vi "AMZ_S3_ERR_Get Call Result.vi"(8 "error in (no error)":errorcluster, 11 "Response body":string) -> (0 "error out":errorcluster, 3 "Call Result":T1)   [LabVIEW 2015, in "LV Interface for Amazon S3.lvlib"]
uses:
  LV Interface for Amazon S3.lvlib
  Typedefs/AMZ_S3_Call Results.ctl
  <vilib>/regexp/Match Regular Expression.xnode
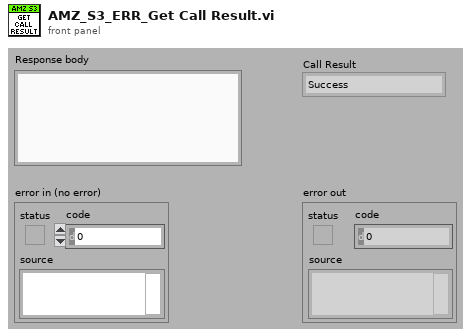
[diagram p1: front panel]
types:
  T1 = typedef "LV Interface for Amazon S3.lvlib/AMZ_S3_Call Results.ctl" = enum16{"Success", "UndefinedError", "AccessDenied", "AccountProblem", "AmbiguousGrantByEmailAddress", "BadDigest", "BucketAlreadyExists", "BucketAlreadyOwnedByYou", "BucketNotEmpty", "CredentialsNotSupported", "CrossLocationLoggingProhibited", "EntityTooSmall", "EntityTooLarge", "ExpiredToken", "IllegalVersioningConfigurationException", "IncompleteBody", "IncorrectNumberOfFilesInPostRequest", "InlineDataTooLarge", "InternalError", "InvalidAccessKeyId", "InvalidAddressingHeader", "InvalidArgument", "InvalidBucketName", "InvalidDigest", "InvalidLocationConstraint", "InvalidPart", "InvalidPartOrder", "InvalidPayer", "InvalidPolicyDocument", "InvalidRange", "InvalidSecurity", "InvalidSOAPRequest", "InvalidStorageClass", "InvalidTargetBucketForLogging", "InvalidToken", "InvalidURI", "KeyTooLong", "MalformedACLError", "MalformedPOSTRequest", "MalformedXML", "MaxMessageLengthExceeded", "MaxPostPreDataLengthExceededError", "MetadataTooLarge", "MethodNotAllowed", "MissingAttachment", "MissingContentLength", "MissingRequestBodyError", "MissingSecurityElement", "MissingSecurityHeader", "NoLoggingStatusForKey", "NoSuchBucket", "NoSuchKey", "NoSuchUpload", "NoSuchVersion", "NotImplemented", "NotSignedUp", "OperationAborted", "PermanentRedirect", "PreconditionFailed", "Redirect", "RequestIsNotMultiPartContent", "RequestTimeout", "RequestTimeTooSkewed", "RequestTorrentOfBucketError", "SignatureDoesNotMatch", "SlowDown", "TemporaryRedirect", "TokenRefreshRequired", "TooManyBuckets", "UnexpectedContent", "UnresolvableGrantByEmailAddress", "UserKeyMustBeSpecified", "LabVIEWError"}
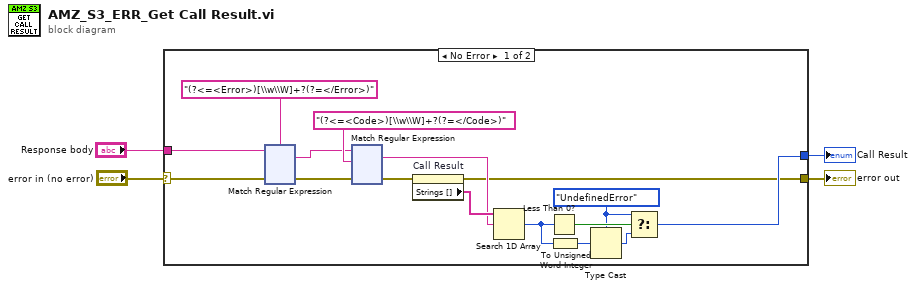
[diagram p0: block diagram]
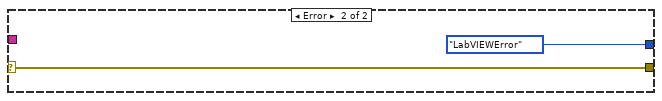
[diagram p2: hidden frame]
diagram:
  n1 = case shown="No Error" "error in (no error)" {
    selector: "error in (no error)" -> [w20 w250]
    tunnel: "Response body" -> [w19 _]
    tunnel: [w5 w250] -> w2
    tunnel: [w10 AMZ_S3_Call_Results."LabVIEWError" ("Call Result")] -> w1
    frame No Error {
      w7 = AMZ_S3_Call_Results."UndefinedError" ("Call Result")
      n2 = xnode "Match Regular Expression"("input string"=w19, "regular expression"="(?<=<Error>)[\\w\\W]+?(?=</Error>)", "error in"=w20) -> ("whole match"=w9:string, "error out"=w17:errorcluster)  [unwired: 3 in, 3 out]
      n3 = xnode "Match Regular Expression"("input string"=w9, "regular expression"="(?<=<Code>)[\\w\\W]+?(?=</Code>)", "error in"=w17) -> ("whole match"=w13:string, "error out"=w15:errorcluster)  [unwired: 3 in, 3 out]
      n4 = property on="Call Result" class="Enum (strict)"(error in=w15) -> (error out=w5:errorcluster, "Strings []"=w14:string[])  [unwired: 1 in, 1 out]
      n5 = Search 1D Array(1D array=w14, element=w13) -> (index of element=w11:i32)  [unwired: 1 in]
      n6 = Less Than 0?(x=w11) -> (x < 0?=w12:bool)
      n7 = To Unsigned Word Integer(number=w11) -> (unsigned 16bit integer=w8:u16)
      n8 = Type Cast(type=w7, x=w8) -> (*(type *) &x=w6:T1)
      n9 = Select(t=w7, s=w12, f=w6) -> (s? t:f=w10:T1)
    }
    frame Error {
    }
  }
  "error out" <- w2
  "Call Result" <- w1
